vi "Set Scroll Bar State).vi"(8 "Error in (No Error)":errorcluster, 10 "Scrollbar Visibility (Always On)":T1(ring), 11 "Pane in":refnum<vi>) -> (0 "Error Out":errorcluster, 3 "Pane Out":refnum<vi>)   [LabVIEW 2024]
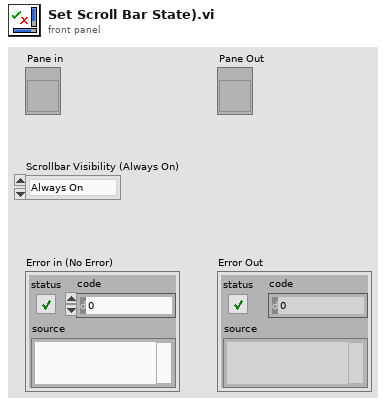
[diagram p1: front panel]
types:
  T1 = enum16{"Always On", "Always Off", "Off While Running"}
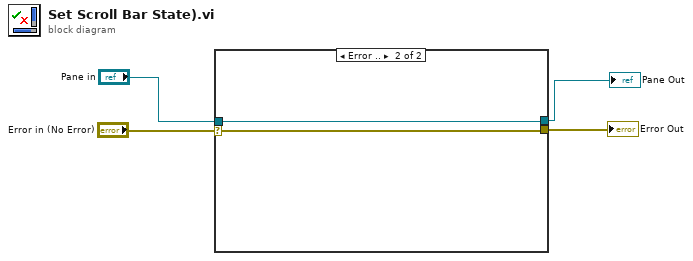
[diagram p0: block diagram]
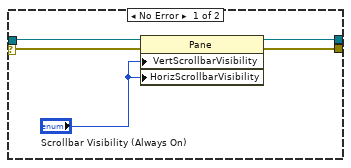
[diagram p2: hidden frame]
diagram:
  n1 = case shown="Error .." "Error in (No Error)" {
    selector: "Error in (No Error)" -> [w5 w10]
    tunnel: "Pane in" -> [w9 w11]
    tunnel: [w7 w10] -> w3
    tunnel: [w6 w11] -> w2
    frame No Error {
      n2 = property on="Property Node" class="Pane"(reference=w9, error in=w5, "VertScrollbarVisibility"="Scrollbar Visibility (Always On)", "HorizScrollbarVisibility"="Scrollbar Visibility (Always On)") -> (reference out=w6:refnum<vi>, error out=w7:errorcluster)
    }
    frame Error {
    }
  }
  "Error Out" <- w3
  "Pane Out" <- w2
